vi "PROJETTTT.vi"(0 "Numérique":i32) -> (1 "Nb cycles":dbl, 2 "Produits Finis":dbl, 3 "Produits defectueux":dbl)   [LabVIEW 2020]
uses:
  lcanneta.ctl
  selector.ctl
panel:
  out "Capteur de présence":bool
  out "Début course":bool
  out "Fin de course":bool
  out "Booléen":bool
  in  "RESET":bool
  in  "stop":bool
  in  "Selector":T1
  out "Glissière":T2 scale=0.0..100.0
  # "STOP"
  # "START"
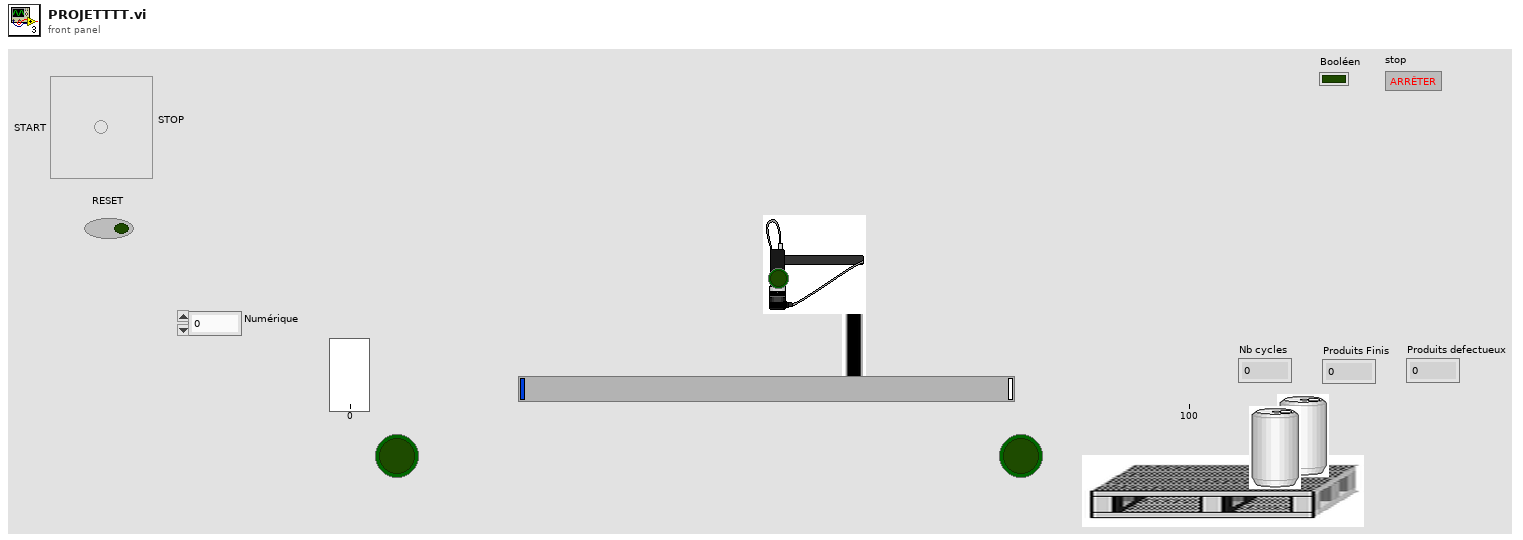
[diagram p1: front panel]
types:
  T1 = typedef "selector.ctl" = bool
  T2 = typedef "lcanneta.ctl" = dbl
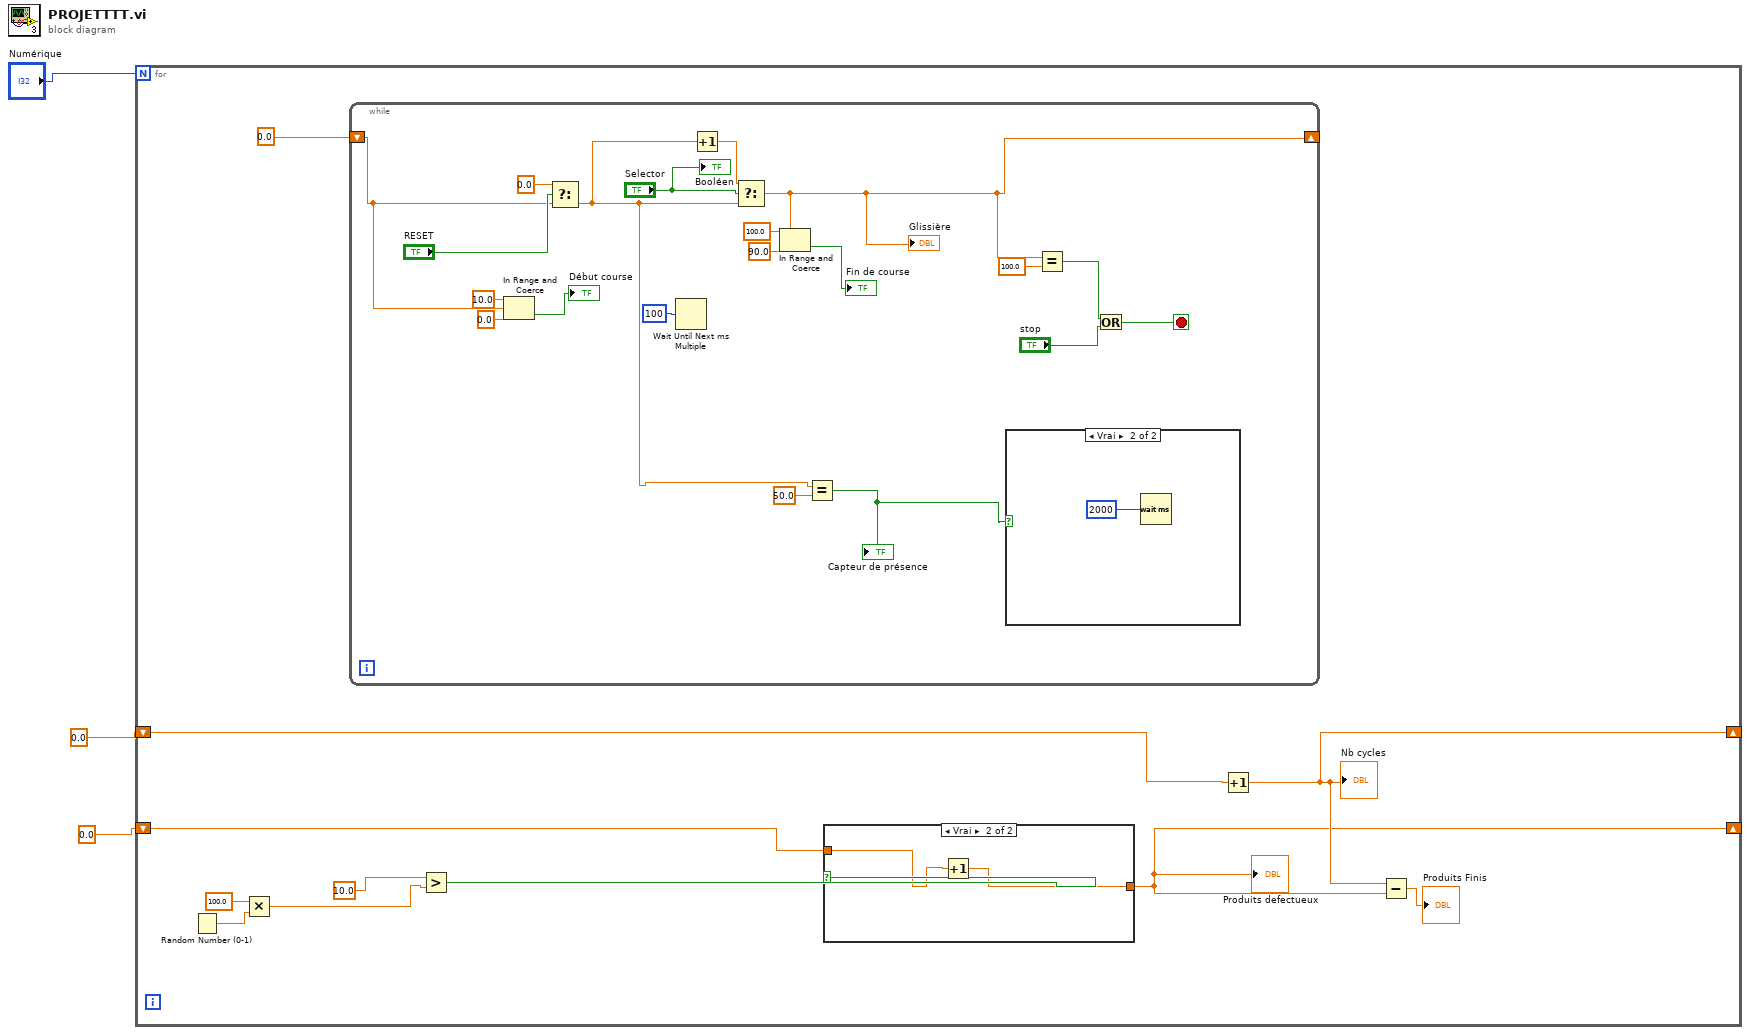
[diagram p0: block diagram]
diagram:
  n1 = for {
    N: "Numérique" -> [_]
    shift-right: [w5] -> _
    shift-left: 0.0 ("x") -> [w13]
    shift-right: [w4] -> _
    shift-left: 0.0 ("x") -> [w7]
    n2 = Random Number (0-1)() -> (number: 0 to 1=w12:dbl)
    n3 = Multiply(x=100.0, y=w12) -> (x*y=w10:dbl)
    n4 = while {
      shift-right: [w19] -> _
      shift-left: 0.0 -> [w27]
      stop <- w22 stop-if-true
      n5 = In Range and Coerce(upper limit=10.0 ("limite supérieure"), x=w27, lower limit=0.0 ("limite inférieure")) -> (In Range?=→"Début course":bool)  [unwired: 1 out]
      n6 = Select(t=0.0 ("cas vrai"), s="RESET", f=w27) -> (s? t:f=w24:dbl)
      n7 = Wait Until Next ms Multiple(millisecond multiple=u32 100 ("n millisecondes")) -> ()  [unwired: 1 out]
      n8 = Increment(x=w24) -> (x+1=w35:dbl)
      n9 = Select(t=w35, s="Selector", f=w24) -> (s? t:f=w19:dbl)
      "Glissière" <- w19
      n10 = In Range and Coerce(upper limit=100.0 ("limite supérieure"), x=w19, lower limit=90.0 ("limite inférieure")) -> (In Range?=→"Fin de course":bool)  [unwired: 1 out]
      n11 = Equal?(x=w24, y=50.0) -> (x = y?=w23:bool)
      "Capteur de présence" <- w23
      n12 = case shown="Vrai" w23 {
        frame False {
        }
        frame True {
          n13 = Wait (ms)(milliseconds to wait=u32 2000 ("valeur de l'horloge en ms")) -> ()  [unwired: 1 out]
        }
      }
      n14 = Equal?(x=w19, y=100.0) -> (x = y?=w18:bool)
      n15 = Or(x=w18, y="stop") -> (x .or. y?=w22:bool)
      "Booléen" <- "Selector"
    }
    n16 = Greater?(x=10.0, y=w10) -> (0:w8:bool)
    n17 = case shown="Vrai" w8 {
      tunnel: w7 -> [w15 w17]
      tunnel: [w15 w16] -> w4
      frame False {
      }
      frame True {
        n18 = Increment(x=w17) -> (x+1=w16:dbl)
      }
    }
    "Produits defectueux" <- w4
    n19 = Increment(x=w13) -> (x+1=w5:dbl)
    "Nb cycles" <- w5
    n20 = Subtract(x=w5, y=w4) -> (x-y=→"Produits Finis":dbl)
  }
